vi "read_file.vi"(3 "error in":errorcluster, 4 "Base directory name":string="trajectories", 5 "File path in":path) -> (0 "error out":errorcluster, 1 "File path out":path, 2 "Trajectory or Scenario read":string)   [LabVIEW 2019]
doc: "Read the trajectory specified from the name or absolute path."
panel:
  # "Trajectory or Scenario Configuration"
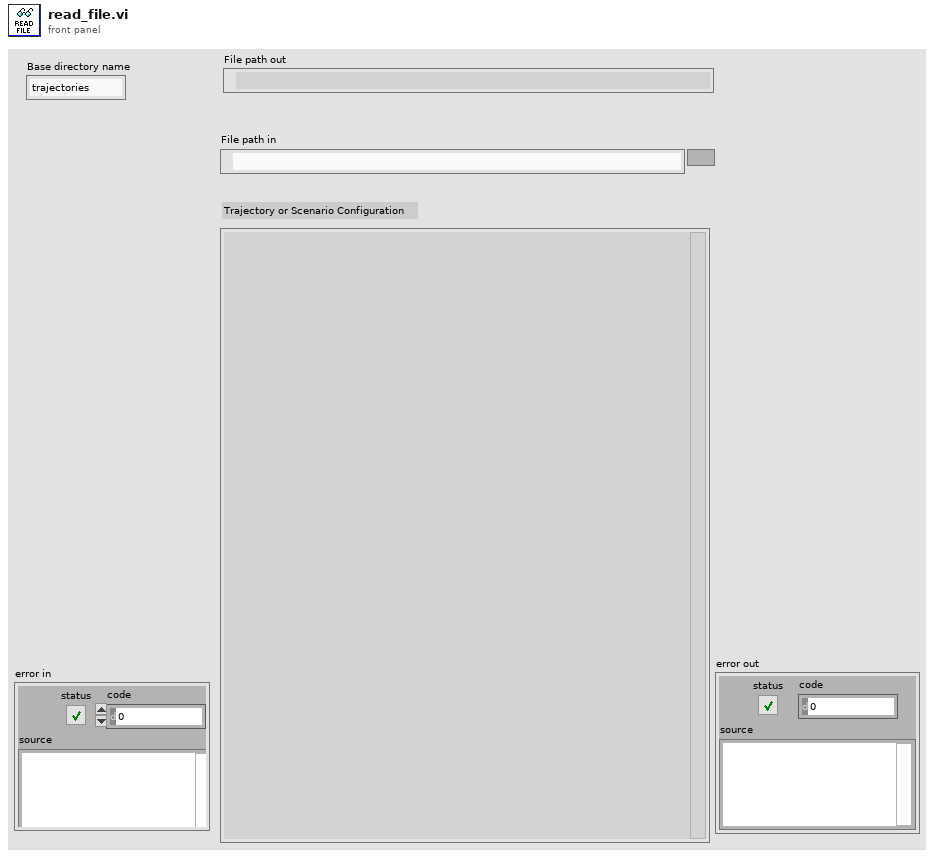
[diagram p1: front panel]
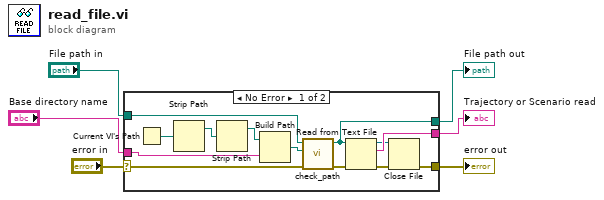
[diagram p0: block diagram]
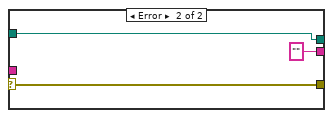
[diagram p2: hidden frame]
diagram:
  n1 = case shown="No Error" "error in" {
    selector: "error in" -> [w12 w22]
    tunnel: [w10 w22] -> w6
    tunnel: [w14 ""] -> w5
    tunnel: "Base directory name" -> [w11 _]
    tunnel: "File path in" -> [w8 w20]
    tunnel: [w7 w20] -> w1
    frame No Error {
      n2 = Current VI's Path() -> (path=w19:path)
      n3 = Strip Path(path=w19) -> (stripped path=w18:path)  [unwired: 1 out]
      n4 = Strip Path(path=w18) -> (stripped path=w17:path)  [unwired: 1 out]
      n5 = Build Path(base path=w17, name or relative path=w11) -> (appended path=w16:path)
      n6 = call "check_path.vi"("error in"=w12, "Base_path"=w16, "Config_Path"=w8) -> ("error out"=w13:errorcluster, "Config_path_out"=w7:path)  [unwired: 3 in]
      n7 = Read from Text File(file (use dialog)=w7, error in=w13) -> (refnum out=w9:refnum<file>, text=w14:string, error out=w15:errorcluster)  [unwired: 2 in, 1 out]
      n8 = Close File(refnum=w9, error in=w15) -> (error out=w10:errorcluster)  [unwired: 1 out]
    }
    frame Error {
    }
  }
  "error out" <- w6
  "Trajectory or Scenario read" <- w5
  "File path out" <- w1
